vi "Actor Core.vi"(8 "error in":errorcluster, 11 "Nested in":refnum<class "User_Console-ATM.lvclass">) -> (0 "error out":errorcluster, 3 "Actor out":refnum<class "Actor.lvclass">)   [LabVIEW 2025, in "User_Console-ATM.lvlib" / "User_Console-ATM.lvclass"]
doc: "(<B>Filename</B>: Actor Framework.lvlib:Actor.lvclass:Actor Core.vi)\n\nReceives messages to the actor, reacts to them, and initiates any error handling that may shut the actor down.\n\nDescendant classes may override this VI to append parallel tasks for the actor to complete while it handles messages. Overrides use the Call Parent Method node."
uses:
  User_Console-ATM.lvclass
  <vilib>/ActorFramework/Actor/Actor.lvclass
  User_Console_States/User_Console_States.lvclass
  <vilib>/ActorFramework/Actor/Actor.lvclass/Actor.ctl
  <vilib>/ActorFramework/Message Enqueuer/Message Enqueuer.lvclass/Message Enqueuer.ctl
  User_Console-ATM.lvclass/User_Console-ATM.ctl
  User_Console_States Messages/update_card_FB Msg/update_card_FB Msg.lvclass/update_card_FB Msg.ctl
  <vilib>/ActorFramework/Message Enqueuer/Init from Existing Queue.vi
  <vilib>/ActorFramework/Message Enqueuer/Enqueue.vi
  User_Console_States Messages/update_card_FB Msg/update_card_FB Msg.lvclass
  <vilib>/ActorFramework/Stop Msg/Stop Msg.lvclass
  <vilib>/ActorFramework/Message Priority Queue/Priority Enqueue.vi
  <vilib>/ActorFramework/Message Enqueuer/Message Enqueuer.lvclass
panel:
  out "Display2":string
  in  "USER CONSOLE :":T1
  in  "TRANSACTIONS:":T2
  in  "Card Reader":bool
  # "USER CONSOLE"
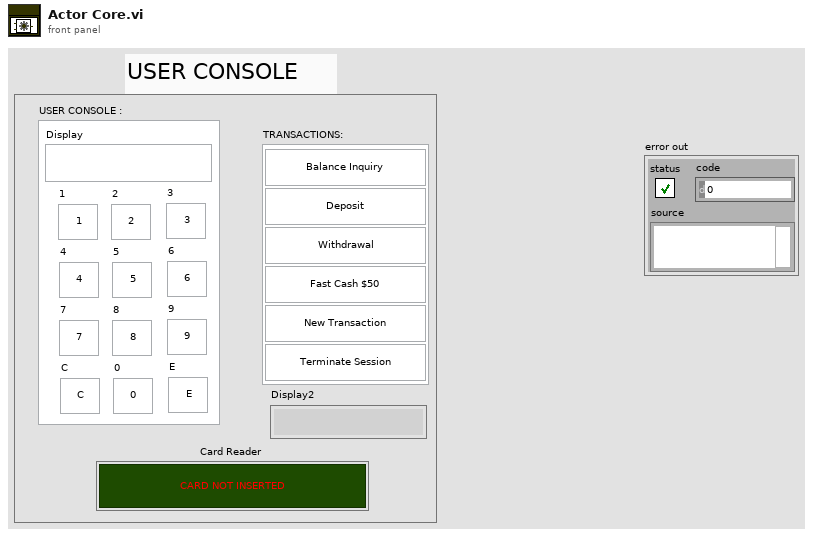
[diagram p1: front panel]
types:
  T1 = cluster{"1":bool, "2":bool, "3":bool, "4":bool, "5":bool, "6":bool, "7":bool, "8":bool, "9":bool, "C":bool, "0":bool, "E":bool, "Display":string}
  T2 = cluster{"Balance Inquiry":bool, "Deposit":bool, "Withdrawal":bool, "Fash Cash $50":bool, "New Transaction":bool, "Terminate Session":bool}
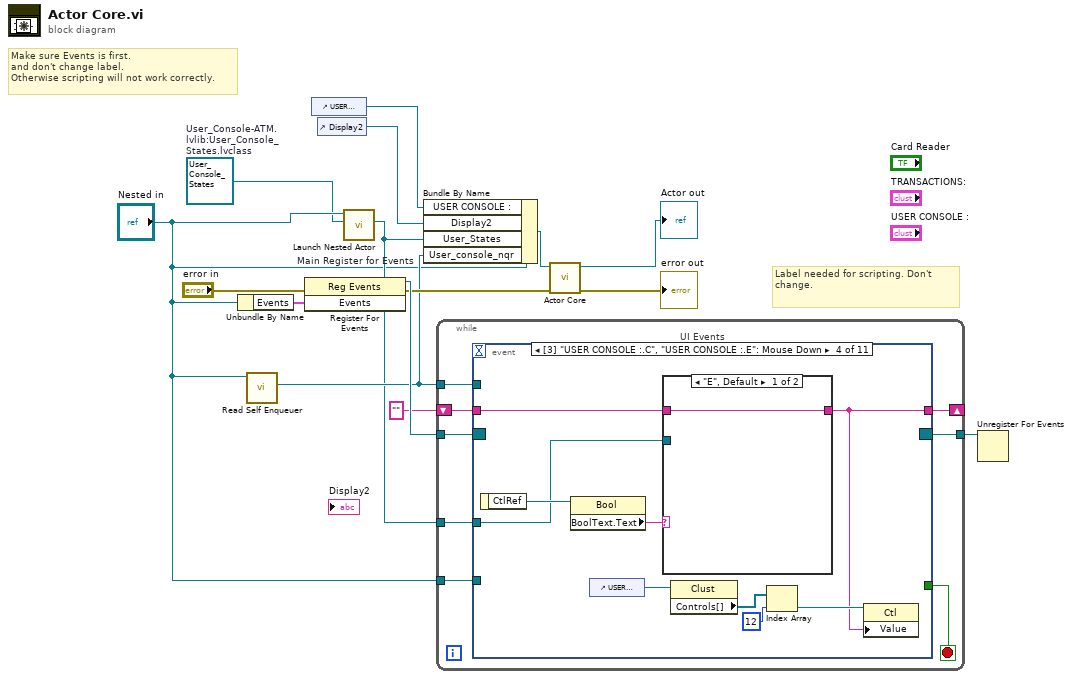
[diagram p0: block diagram]
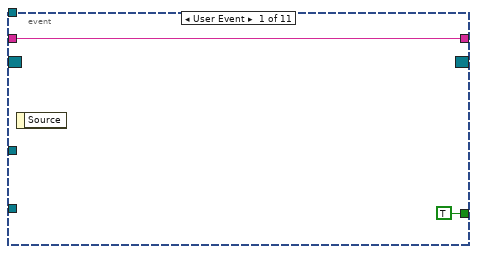
[diagram p2: hidden frame]
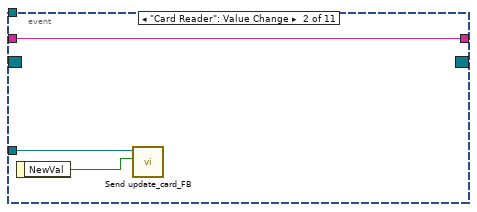
[diagram p3: hidden frame]
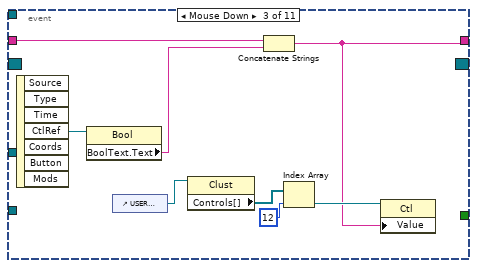
[diagram p4: hidden frame]
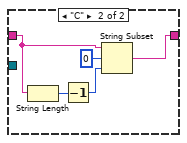
[diagram p5: hidden frame]
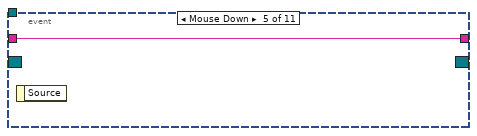
[diagram p6: hidden frame]
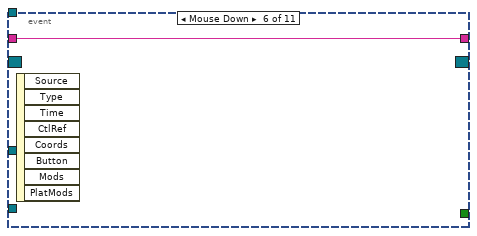
[diagram p7: hidden frame]
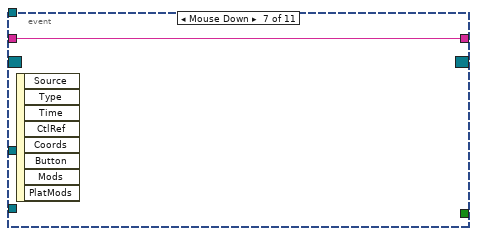
[diagram p8: hidden frame]
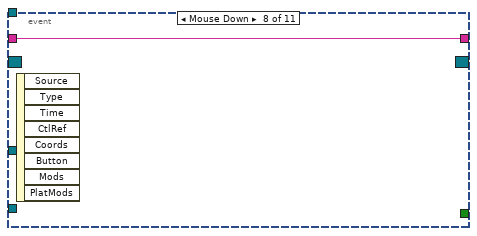
[diagram p9: hidden frame]
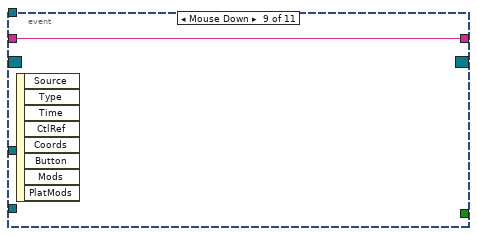
[diagram p10: hidden frame]
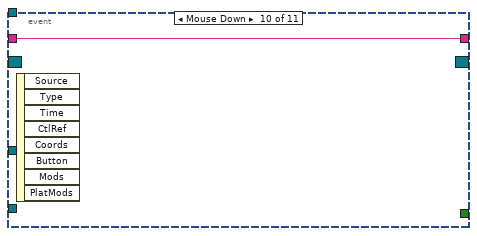
[diagram p11: hidden frame]
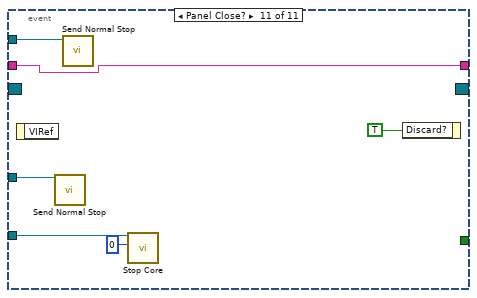
[diagram p12: hidden frame]
diagram:
  w1 = refnum<class "User_Console_States.lvclass"> refnum  # User_Console-ATM.lvlib:User_Console_States.lvclass
  # "Label needed for scripting. Don't change."
  # "Make sure Events is first.\nand don't change label.\nOtherwise scripting will not work correctly."
  n1 = Unbundle By Name("Nested in") -> ("Events"=w12:cluster{"Stop":refnum<user-event>})
  n2 = call <vilib>:"Read Self Enqueuer.vi"("Actor"="Nested in") -> ("Self Enqueuer"=w6:refnum<class "Message Enqueuer.lvclass">)  [unwired: 10 in]
  n3 = register-events "Main Register for Events"(error in="error in", w12) -> (reference out=w13:refnum<event-registration>, error out=w9:errorcluster)  [unwired: 1 in]
  n4 = control-ref of="USER CONSOLE :"() -> (w4:refnum<vi>)
  n5 = control-ref of="Display2"() -> (w7:refnum<vi>)
  n6 = call <vilib>:"Launch Nested Actor.vi"("Nested Actor"=w1, "Caller Actor in"="Nested in") -> ("Nested Actor's Enqueuer"=w3:refnum<class "Message Enqueuer.lvclass">)  [unwired: 7 in, 2 out]
  n7 = Bundle By Name(cluster="Nested in", "USER CONSOLE :"=w4, "Display2"=w7, "User_States"=w3, "User_console_nqr"=w6) -> (w8:refnum<class "User_Console-ATM.lvclass">)
  n8 = while {
    tunnel: w13 -> [w23]
    tunnel: [w21] -> w11
    tunnel: w6 -> [w20]
    shift-right: [w18] -> _
    shift-left: "" -> [w19]
    tunnel: w3 -> [w17]
    tunnel: "Nested in" -> [w16]
    stop <- w22 stop-if-true
    n9 = event "UI Events" shown="[3] \"USER CONSOLE :.C\", \"USER CONSOLE :.E\": Mouse Down" {
      selector: w23 -> [_ _ _ _ _ _ _ _ _ _ _]
      dyn-events: [_ _ _ _ _ _ _ _ _ _ _] -> w21
      timeout: _ -> [_ _ _ _ _ _ _ _ _ _ _]
      tunnel: [TRUE _ _ _ _ _ _ _ _ _ _] -> w22
      tunnel: w20 -> [_ _ _ _ _ _ _ _ _ _ w62]
      tunnel: w19 -> [w24 w28 w35 w43 w52 w53 w54 w55 w56 w57 w61]
      tunnel: [w24 w28 w29 w39 w52 w53 w54 w55 w56 w57 w61] -> w18
      tunnel: w17 -> [_ w27 _ w37 _ _ _ _ _ _ w60]
      tunnel: w16 -> [_ _ _ _ _ _ _ _ _ _ w59]
      event User Event {
        n10 = event-data() -> ()  [unwired: 1 in, 1 out]
      }
      event "Card Reader": Value Change {
        n11 = event-data() -> ("NewVal"=w26:bool)  [unwired: 1 in]
        n12 = call "Send update_card_FB.vi"("Card"=w26, "Message Enqueuer"=w27) -> ()  [unwired: 8 in, 2 out]
      }
      event "USER CONSOLE :.1", "USER CONSOLE :.2", "USER CONSOLE :.3", "USER CONSOLE :.4", "USER CONSOLE :.5", "USER CONSOLE :.6", "USER CONSOLE :.7", "USER CONSOLE :.8", "USER CONSOLE :.9", "USER CONSOLE :.0": Mouse Down {
        n13 = event-data() -> ("CtlRef"=w36:refnum<vi>)  [unwired: 1 in, 6 out]
        n14 = property class="Bool"(reference=w36) -> ("BoolText.Text"=w34:string)  [unwired: 1 in, 2 out]
        n15 = control-ref of="USER CONSOLE :"() -> (w33:refnum<vi>)
        n16 = property class="Clust"(reference=w33) -> ("Controls[]"=w32:refnum<vi>[])  [unwired: 1 in, 2 out]
        n17 = Concatenate Strings(w35, w34) -> (w29:string)
        n18 = Index Array(array=w32, index=12) -> (element=w30:refnum<vi>)
        n19 = property class="Ctl"(reference=w30, "Value"=w29) -> ()  [unwired: 1 in, 2 out]
      }
      event "USER CONSOLE :.C", "USER CONSOLE :.E": Mouse Down {
        n20 = event-data() -> ("CtlRef"=w45:refnum<vi>)  [unwired: 1 in]
        n21 = property class="Bool"(reference=w45) -> ("BoolText.Text"=w44:string)  [unwired: 1 in, 2 out]
        n22 = control-ref of="USER CONSOLE :"() -> (w38:refnum<vi>)
        n23 = case shown="\"E\", Default" w44 {
          tunnel: w43 -> [w46 w50]
          tunnel: [w46 w48] -> w39
          tunnel: w37 -> [_ _]
          frame "E", Default {
          }
          frame "C" {
            n24 = String Length(string=w50) -> (length=w51:i32)
            n25 = Decrement(x=w51) -> (x-1=w49:i32)
            n26 = String Subset(string=w50, offset (0)=0, length (rest)=w49) -> (substring=w48:string)
          }
        }
        n27 = property class="Clust"(reference=w38) -> ("Controls[]"=w42:refnum<vi>[])  [unwired: 1 in, 2 out]
        n28 = Index Array(array=w42, index=12) -> (element=w40:refnum<vi>)
        n29 = property class="Ctl"(reference=w40, "Value"=w39) -> ()  [unwired: 1 in, 2 out]
      }
      event "TRANSACTIONS:.Balance Inquiry": Mouse Down {
        n30 = event-data() -> ()  [unwired: 1 in, 1 out]
      }
      event "TRANSACTIONS:.Deposit": Mouse Down {
        n31 = event-data() -> ()  [unwired: 1 in, 8 out]
      }
      event "TRANSACTIONS:.Withdrawal": Mouse Down {
        n32 = event-data() -> ()  [unwired: 1 in, 8 out]
      }
      event "TRANSACTIONS:.Fash Cash $50": Mouse Down {
        n33 = event-data() -> ()  [unwired: 1 in, 8 out]
      }
      event "TRANSACTIONS:.New Transaction": Mouse Down {
        n34 = event-data() -> ()  [unwired: 1 in, 8 out]
      }
      event "TRANSACTIONS:.Terminate Session": Mouse Down {
        n35 = event-data() -> ()  [unwired: 1 in, 8 out]
      }
      event Panel Close? {
        n36 = event-data() -> ()  [unwired: 1 in, 1 out]
        n37 = call <vilib>:"Send Normal Stop.vi"("Message Enqueuer"=w60) -> ()  [unwired: 10 in, 1 out]
        n38 = call <vilib>:"Send Normal Stop.vi"("Message Enqueuer"=w62) -> ()  [unwired: 10 in, 1 out]
        n39 = call-dynamic "Stop Core.vi"("final error code"=0, "Nested in"=w59) -> ()  [unwired: 9 in, 1 out]
        n40 = event-data("Discard?"=TRUE) -> ()  [unwired: 1 in, 1 out]
      }
    }
  }
  n41 = call-parent "Actor Core.vi"("error in"=w9, "Actor in"=w8) -> ("error out"=→"error out":errorcluster, "Actor out"=→"Actor out":refnum<class "Actor.lvclass">)  [unwired: 8 in]
  n42 = Unregister For Events(event registration refnum=w11) -> ()  [unwired: 1 in, 1 out]
